vi "Main.vi"() -> ()   [LabVIEW 2017, in "WebServiceImporter.lvlib" / "Main Panel.lvlib" / "Input Info.lvlib"]
uses:
  <vilib>/Platform/WebService/Main Panel/Pages/Input Info/Input Info.lvlib
  <vilib>/Platform/WebService/Global/Const Strings.vi
  <vilib>/Platform/WebService/Main Panel/Pages/Input Info/Events/Events.lvlib
  <vilib>/Platform/WebService/Main Panel/Events/Events.lvlib
  <vilib>/Platform/WebService/Main Panel/Pages/Preview/Preview.lvlib
  <vilib>/Platform/WebService/ProxyDll Generator/ProxyDll Generator.lvlib
  <vilib>/Platform/WebService/VI Generator/VI Generator.lvlib
  <vilib>/Platform/WebService/Error Handling/Error Handling.lvlib
  <vilib>/Platform/WebService/Main Panel/Main Panel.lvlib
  <vilib>/Platform/WebService/WebServiceImporter.lvlib
panel:
  in  "Panel":enum32{"Interface Frame", "Hidden Controls"}(tab)
  out "Error Message":string="SOAP protocol is not detected. We only support service using SOAP."
  in  "Destination Directory":path
  in  "Project Library Name (.lvlib)":string
  out "File name warning":string="A library name cannot contain any of the following characters.\n\\ / : * ? \" < > |"
  # "Input the project library and destination directory"
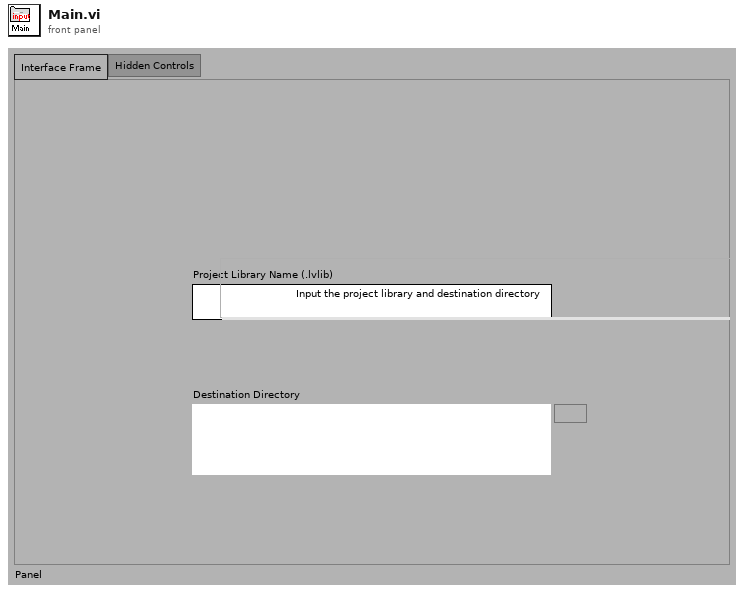
[diagram p1: front panel]
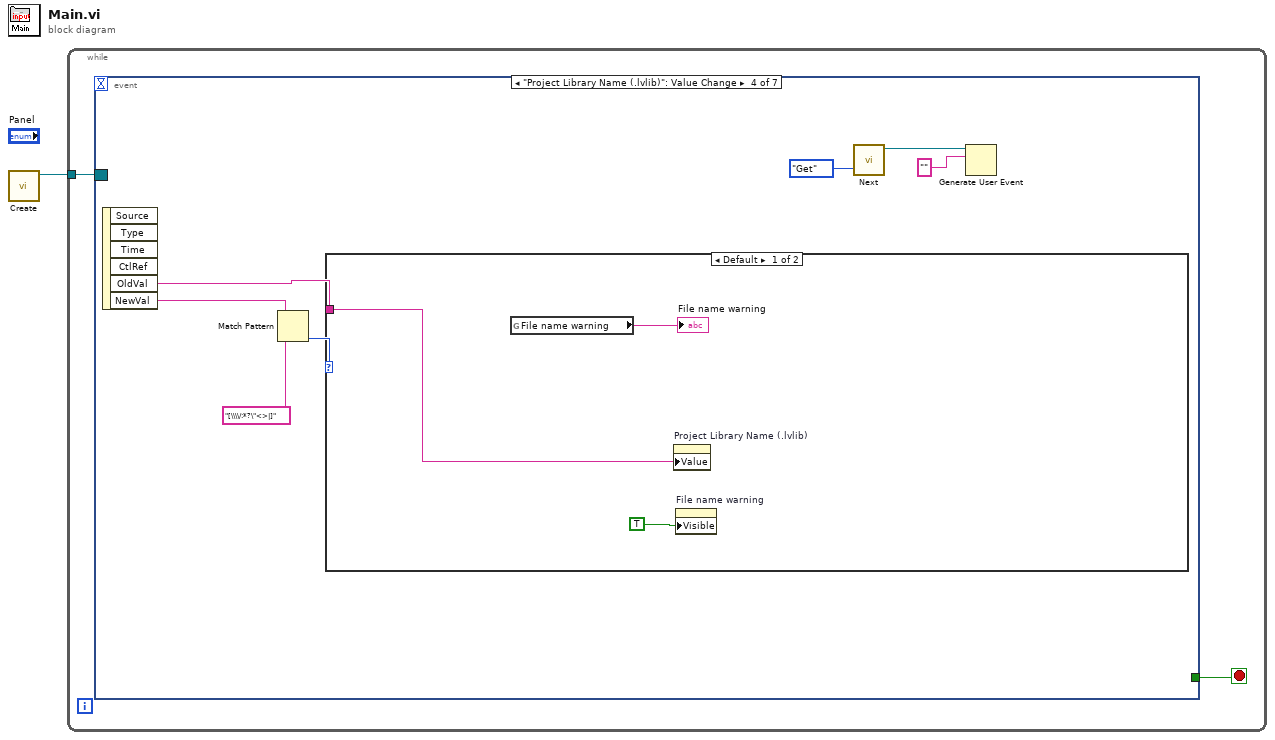
[diagram p0: block diagram]
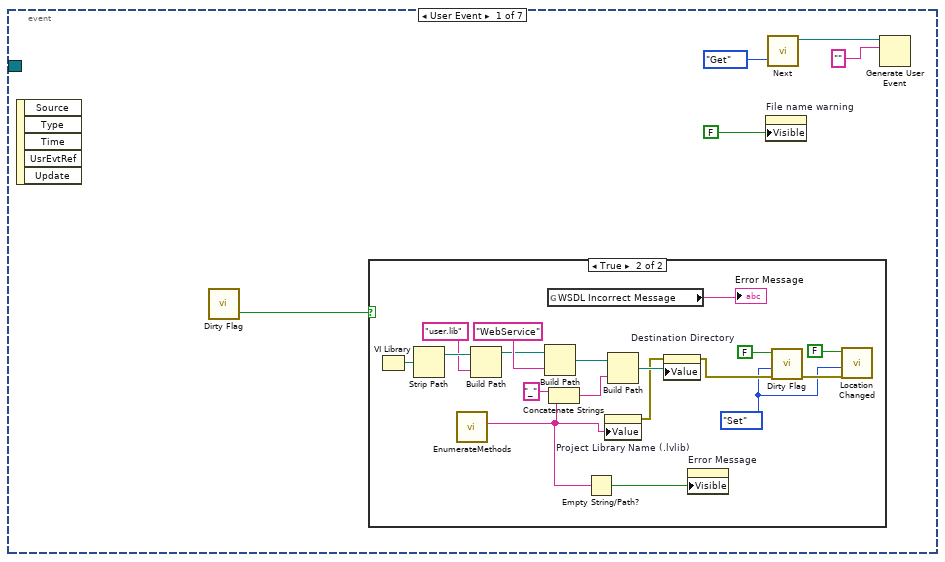
[diagram p2: hidden frame]
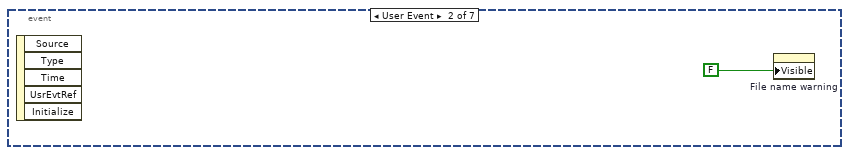
[diagram p4: hidden frame]
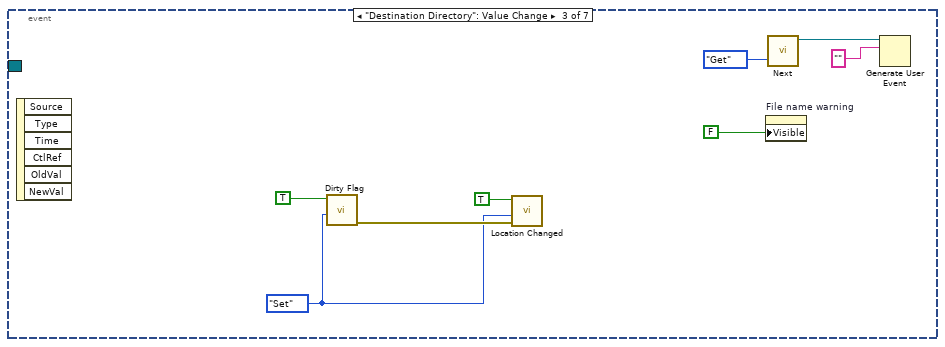
[diagram p5: hidden frame]
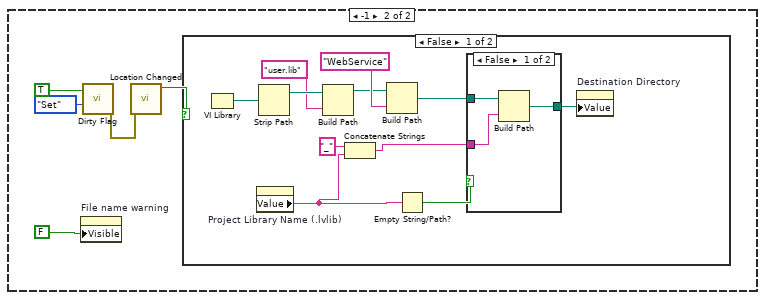
[diagram p6: hidden frame]
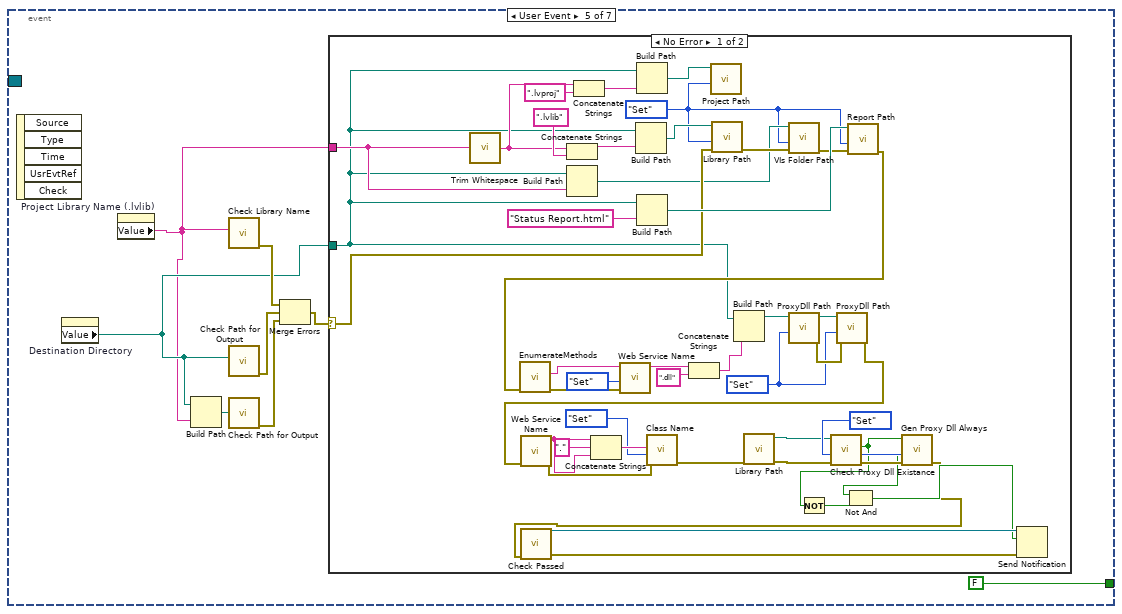
[diagram p9: hidden frame]
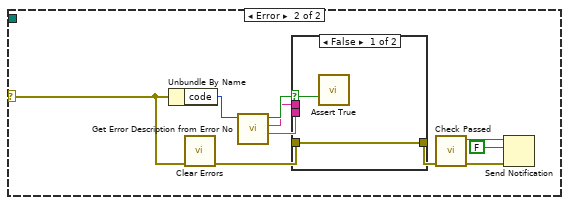
[diagram p10: hidden frame]
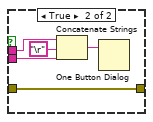
[diagram p11: hidden frame]
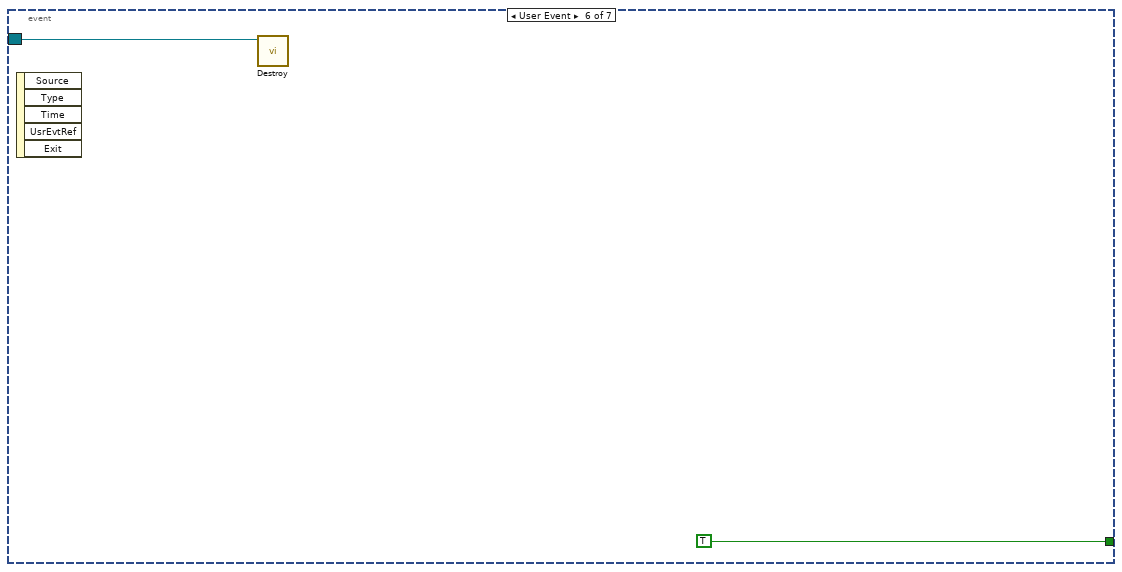
[diagram p12: hidden frame]
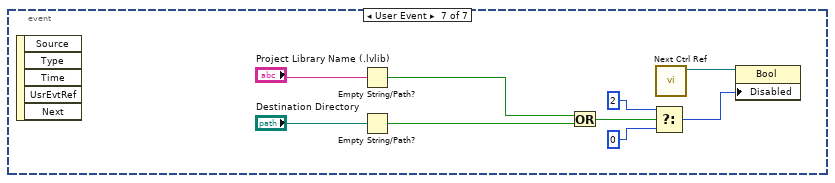
[diagram p13: hidden frame]
diagram:
  n1 = call <vilib>:"Create.vi"() -> ("Event Registration Refnum"=w1:refnum<event-registration>)  [unwired: 1 in, 10 out]
  n2 = while {
    tunnel: w1 -> [w3]
    stop <- w2 stop-if-true
    n3 = event shown="[3] \"Project Library Name (.lvlib)\": Value Change" {
      selector: w3 -> [_ _ _ _ _ w137 _]
      dyn-events: _ -> [_ _ _ _ _ _ _]
      timeout: _ -> [_ _ _ _ _ _ _]
      tunnel: [_ _ _ _ FALSE TRUE _] -> w2
      event User Event {
        n4 = event-data() -> ()  [unwired: 6 out]
        n5 = call <vilib>:"Dirty Flag.vi"() -> ("Dirty (out)"=w8:bool)  [unwired: 3 in, 8 out]
        n6 = case shown="True" w8 {
          frame False {
          }
          frame True {
            w15 = enum16{"Get", "Set"}."Set" ("Operation")
            n7 = VI Library() -> (path=w25:path)
            n8 = Strip Path(path=w25) -> (stripped path=w24:path)  [unwired: 1 out]
            n9 = call <vilib>:"EnumerateMethods.vi"() -> ("Service Name"=w11:string)  [unwired: 1 in, 10 out]
            n10 = Build Path(base path=w24, name or relative path="user.lib") -> (appended path=w22:path)
            n11 = Build Path(base path=w22, name or relative path="WebService") -> (appended path=w21:path)
            n12 = global read "Const Strings.vi" "WSDL Incorrect Message"() -> (→"Error Message":string)
            n13 = Concatenate Strings("_" ("string"), w11) -> (w12:string)
            n14 = Empty String/Path?(string/path=w11) -> (empty?=w10:bool)
            n15 = property on="Project Library Name (.lvlib)" class="Str"("Value"=w11) -> (error out=w19:errorcluster)  [unwired: 2 in, 1 out]
            n16 = Build Path(base path=w21, name or relative path=w12) -> (appended path=w20:path)
            n17 = property on="Destination Directory" class="Path"(error in=w19, "Value"=w20) -> (error out=w18:errorcluster)  [unwired: 1 in, 1 out]
            n18 = property on="Error Message" class="Str"("Visible"=w10) -> ()  [unwired: 2 in, 2 out]
            n19 = call <vilib>:"Dirty Flag.vi"("error in (no error)"=w18, "Operation"=w15, "Dirty"=FALSE) -> ("error out"=w16:errorcluster)  [unwired: 8 out]
            n20 = call <vilib>:"Location Changed.vi"("error in (no error)"=w16, "Operation"=w15, "Location Changed"=FALSE) -> ()  [unwired: 9 out]
          }
        }
        n21 = property on="File name warning" class="Str"("Visible"=FALSE) -> ()  [unwired: 2 in, 2 out]
        n22 = call <vilib>:"Next.vi"("Operation"=enum16{"Get", "Set"}."Get") -> ("user event (out)"=w5:refnum<user-event>)  [unwired: 1 in, 9 out]
        n23 = Generate User Event(user event=w5, event data cluster="" ("event data")) -> ()  [unwired: 2 in, 2 out]
      }
      event User Event {
        n24 = event-data() -> ()  [unwired: 6 out]
        n25 = property on="File name warning" class="Str"("Visible"=FALSE) -> ()  [unwired: 2 in, 2 out]
      }
      event "Destination Directory": Value Change {
        w33 = enum16{"Get", "Set"}."Set" ("Operation")
        n26 = event-data() -> ()  [unwired: 7 out]
        n27 = call <vilib>:"Dirty Flag.vi"("Operation"=w33, "Dirty"=TRUE) -> ("error out"=w34:errorcluster)  [unwired: 1 in, 8 out]
        n28 = call <vilib>:"Location Changed.vi"("error in (no error)"=w34, "Operation"=w33, "Location Changed"=TRUE) -> ()  [unwired: 9 out]
        n29 = property on="File name warning" class="Str"("Visible"=FALSE) -> ()  [unwired: 2 in, 2 out]
        n30 = call <vilib>:"Next.vi"("Operation"=enum16{"Get", "Set"}."Get") -> ("user event (out)"=w29:refnum<user-event>)  [unwired: 1 in, 9 out]
        n31 = Generate User Event(user event=w29, event data cluster="" ("event data")) -> ()  [unwired: 2 in, 2 out]
      }
      event "Project Library Name (.lvlib)": Value Change {
        n32 = event-data() -> ("OldVal"=w36:string, "NewVal"=w39:string)  [unwired: 5 out]
        n33 = Match Pattern(string=w39, regular expression="[\\\\/:*?\"<>|]") -> (offset past match=w38:i32)  [unwired: 4 out]
        n34 = case shown="Default" w38 {
          tunnel: w36 -> [w45 _]
          frame Default {
            n35 = global read "Const Strings.vi" "File name warning"() -> (→"File name warning":string)
            n36 = property on="Project Library Name (.lvlib)" class="Str"("Value"=w45) -> ()  [unwired: 2 in, 2 out]
            n37 = property on="File name warning" class="Str"("Visible"=TRUE) -> ()  [unwired: 2 in, 2 out]
          }
          frame -1 {
            n38 = property on="File name warning" class="Str"("Visible"=FALSE) -> ()  [unwired: 2 in, 2 out]
            n39 = call <vilib>:"Dirty Flag.vi"("Operation"=enum16{"Get", "Set"}."Set", "Dirty"=TRUE) -> ("error out"=w48:errorcluster)  [unwired: 1 in, 8 out]
            n40 = call <vilib>:"Location Changed.vi"("error in (no error)"=w48) -> ("Location Changed 2"=w47:bool)  [unwired: 2 in, 8 out]
            n41 = case shown="False" w47 {
              frame False {
                n42 = VI Library() -> (path=w60:path)
                n43 = property on="Project Library Name (.lvlib)" class="Str"() -> ("Value"=w51:string)  [unwired: 2 in, 2 out]
                n44 = Strip Path(path=w60) -> (stripped path=w59:path)  [unwired: 1 out]
                n45 = Build Path(base path=w59, name or relative path="user.lib") -> (appended path=w57:path)
                n46 = Concatenate Strings("_" ("string"), w51) -> (w52:string)
                n47 = Build Path(base path=w57, name or relative path="WebService") -> (appended path=w56:path)
                n48 = Empty String/Path?(string/path=w51) -> (empty?=w54:bool)
                n49 = case shown="False" w54 {
                  tunnel: w56 -> [w64 w65]
                  tunnel: w52 -> [w63 _]
                  tunnel: [w62 w65] -> w55
                  frame False {
                    n50 = Build Path(base path=w64, name or relative path=w63) -> (appended path=w62:path)
                  }
                  frame True {
                  }
                }
                n51 = property on="Destination Directory" class="Path"("Value"=w55) -> ()  [unwired: 2 in, 2 out]
              }
              frame True {
              }
            }
          }
        }
        n52 = call <vilib>:"Next.vi"("Operation"=enum16{"Get", "Set"}."Get") -> ("user event (out)"=w40:refnum<user-event>)  [unwired: 1 in, 9 out]
        n53 = Generate User Event(user event=w40, event data cluster="" ("event data")) -> ()  [unwired: 2 in, 2 out]
      }
      event User Event {
        n54 = event-data() -> ()  [unwired: 6 out]
        n55 = property on="Destination Directory" class="Path"() -> ("Value"=w68:path)  [unwired: 2 in, 2 out]
        n56 = property on="Project Library Name (.lvlib)" class="Str"() -> ("Value"=w66:string)  [unwired: 2 in, 2 out]
        n57 = Build Path(base path=w68, name or relative path=w66) -> (appended path=w69:path)
        n58 = call <vilib>:"Check Library Name.vi"("Library Name"=w66) -> ("error out"=w73:errorcluster)  [unwired: 1 in, 9 out]
        n59 = call <vilib>:"Check Path for Output.vi"("Path"=w68) -> ("error out"=w72:errorcluster)  [unwired: 1 in, 9 out]
        n60 = call <vilib>:"Check Path for Output.vi"("Path"=w69) -> ("error out"=w70:errorcluster)  [unwired: 1 in, 9 out]
        n61 = Merge Errors(w73, w72, w70) -> (w71:errorcluster)
        n62 = case shown="No Error" w71 {
          selector: w71 -> [w97 w120]
          tunnel: w66 -> [w92 _]
          tunnel: w68 -> [w87 _]
          frame No Error {
            w86 = enum16{"Get", "Set"}."Set" ("Op")
            w111 = enum16{"Get", "Set"}."Set" ("Operation")
            n63 = call <vilib>:"Trim Whitespace.vi"("string"=w92) -> ("trimmed string"=w90:string)  [unwired: 1 in]
            n64 = Concatenate Strings(w90, ".lvlib" ("string")) -> (w107:string)
            n65 = Build Path(base path=w87, name or relative path=w92) -> (appended path=w91:path)
            n66 = Concatenate Strings(w90, ".lvproj" ("string")) -> (w88:string)
            n67 = Build Path(base path=w87, name or relative path=w107) -> (appended path=w106:path)
            n68 = Build Path(base path=w87, name or relative path=w88) -> (appended path=w85:path)
            n69 = Build Path(base path=w87, name or relative path="Status Report.html") -> (appended path=w109:path)
            n70 = call <vilib>:"Project Path.vi"("Operation"=w86, "Path"=w85) -> ()  [unwired: 1 in, 9 out]
            n71 = call <vilib>:"Library Path.vi"("error in (no error)"=w97, "Operation"=w86, "Path"=w106) -> ("error out"=w95:errorcluster)  [unwired: 8 out]
            n72 = call <vilib>:"VIs Folder Path.vi"("error in (no error)"=w95, "Operation"=w86, "Path"=w91) -> ("error out"=w94:errorcluster)  [unwired: 8 out]
            n73 = call <vilib>:"Report Path.vi"("error in (no error)"=w94, "Op"=w86, "Path"=w109) -> ("error out"=w96:errorcluster)  [unwired: 8 out]
            n74 = call <vilib>:"EnumerateMethods.vi"("error in (no error)"=w96) -> ("error out"=w105:errorcluster, "Service Name"=w103:string)  [unwired: 9 out]
            n75 = call <vilib>:"Web Service Name.vi"("error in (no error)"=w105, "Operation"=enum16{"Get", "Set"}."Set", "Web Service Name"=w103) -> ("Web Service Name (out)"=w116:string)  [unwired: 8 out]
            n76 = Concatenate Strings(w116, ".dll") -> (w114:string)
            n77 = Build Path(base path=w87, name or relative path=w114) -> (appended path=w115:path)
            n78 = call <vilib>:"ProxyDll Path.vi"("Operation"=w111, "ProxyDll Path"=w115) -> ("error out"=w112:errorcluster, "ProxyDll Path (out)"=w113:path)  [unwired: 1 in, 7 out]
            n79 = call <vilib>:"ProxyDll Path.vi"("error in (no error)"=w112, "Operation"=w111, "ProxyDll Path"=w113) -> ("error out"=w98:errorcluster)  [unwired: 8 out]
            n80 = call <vilib>:"Web Service Name.vi"("error in (no error)"=w98) -> ("error out"=w100:errorcluster, "Web Service Name (out)"=w74:string)  [unwired: 2 in, 7 out]
            n81 = Concatenate Strings(w74, "." ("string"), w74) -> (w101:string)
            n82 = call <vilib>:"Class Name.vi"("error in (no error)"=w100, "Operation"=enum16{"Get", "Set"}."Set", "Class Name"=w101) -> ("error out"=w75:errorcluster)  [unwired: 8 out]
            n83 = call <vilib>:"Library Path.vi"("error in (no error)"=w75) -> ("error out"=w80:errorcluster, "Path (out)"=w79:path)  [unwired: 2 in, 7 out]
            n84 = call <vilib>:"Check Proxy Dll Existance.vi"("error in (no error)"=w80, "Proxy Dll Path"=w79) -> ("error out"=w82:errorcluster, "Existing?"=w78:bool, "Overwrite?"=w77:bool)  [unwired: 7 out]
            n85 = Not(x=w77) -> (.not. x?=w76:bool)
            n86 = Not And(1:w76, 2:w78) -> (0:w84:bool)
            n87 = call <vilib>:"Gen Proxy Dll Always.vi"("error in (no error)"=w82, "Operation"=enum16{"Get", "Set"}."Set", "Generate whatever"=w77) -> ("error out"=w83:errorcluster)  [unwired: 8 out]
            n88 = call <vilib>:"Check Passed.vi"("error in (no error)"=w83) -> ("error out"=w110:errorcluster, "notifier  (out)"=w118:refnum<notifier>)  [unwired: 2 in, 7 out]
            n89 = Send Notification(notification=w84, notifier=w118, error in (no error)=w110) -> ()  [unwired: 2 out]
          }
          frame Error {
            n90 = Unbundle By Name(w120) -> ("code"=w126:i32)
            n91 = call <vilib>:"Clear Errors.vi"("error in (no error)"=w120) -> ("error out"=w119:errorcluster)  [unwired: 1 in, 5 out]
            n92 = call <vilib>:"Get Error Description from Error No.vi"("Error Number"=w126) -> ("Error Description"=w123:string, "Error Title"=w124:string, "Found?"=w125:bool)  [unwired: 8 out]
            n93 = case shown="False" w125 {
              selector: w125 -> [w130 _]
              tunnel: w124 -> [_ w135]
              tunnel: w123 -> [_ w133]
              tunnel: w119 -> [w129 w131]
              tunnel: [w129 w131] -> w122
              frame False {
                n94 = call <vilib>:"Assert True.vi"("Boolean ( True)"=w130) -> ()  [unwired: 11 out]
              }
              frame True {
                n95 = Concatenate Strings(w135, "\r", w133) -> (w132:string)
                n96 = One Button Dialog(message=w132) -> ()  [unwired: 2 out]
              }
            }
            n97 = call <vilib>:"Check Passed.vi"("error in (no error)"=w122) -> ("error out"=w121:errorcluster, "notifier  (out)"=w127:refnum<notifier>)  [unwired: 2 in, 7 out]
            n98 = Send Notification(notification=FALSE, notifier=w127, error in (no error)=w121) -> ()  [unwired: 2 out]
          }
        }
      }
      event User Event {
        n99 = event-data() -> ()  [unwired: 6 out]
        n100 = call <vilib>:"Destroy.vi"("Event Registration Refnum"=w137) -> ()  [unwired: 1 in, 10 out]
      }
      event User Event {
        n101 = event-data() -> ()  [unwired: 6 out]
        n102 = Empty String/Path?(string/path="Project Library Name (.lvlib)") -> (empty?=w145:bool)
        n103 = Empty String/Path?(string/path="Destination Directory") -> (empty?=w144:bool)
        n104 = Or(x=w145, y=w144) -> (x .or. y?=w146:bool)
        n105 = Select(t=u8 2 ("Disabled"), s=w146, f=u8 0 ("Disabled")) -> (s? t:f=w141:u8)
        n106 = call <vilib>:"Next Ctrl Ref.vi"() -> ("Ctl Refnum (out)"=w138:refnum<vi>)  [unwired: 3 in, 8 out]
        n107 = property class="Bool"(reference=w138, "Disabled"=w141) -> ()  [unwired: 1 in, 2 out]
      }
    }
  }
